vi "Calculate_Desired_Flowrates.vi"(8 "Strength (% by volume)":dbl=3.0 format="%.2f", 9 "Carrier_2 Q (l/min)":dbl=20.0 format="%.2f", 10 "Carrier_1 Q (l/min)":dbl=20.0 format="%.2f") -> (0 "Error Message":string, 1 "Trace Q l/min":dbl format="%.2f", 2 "Carrier 2 l/min":dbl format="%.2f", 3 "Carrier 1 l/min":dbl format="%.2f", 4 "Carrier Info":string)   [LabVIEW 2014]
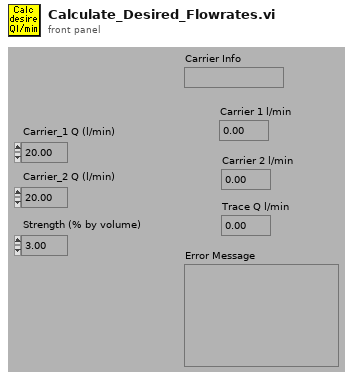
[diagram p1: front panel]
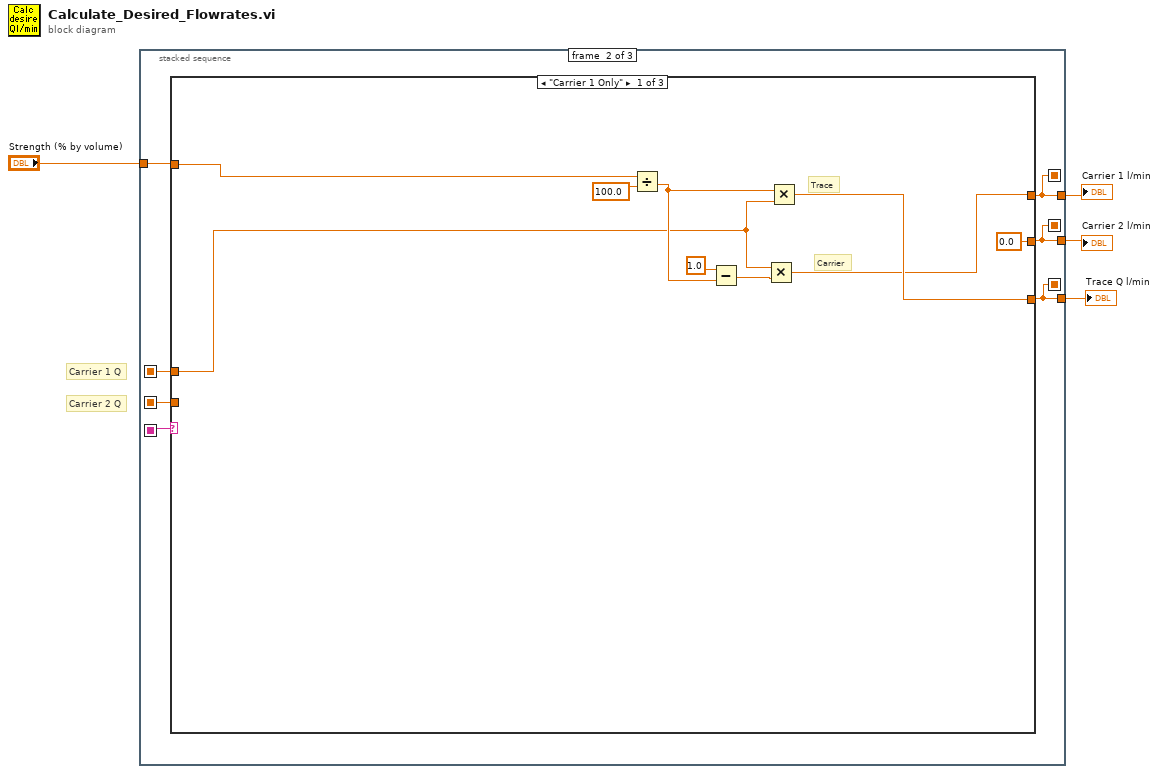
[diagram p0: block diagram]
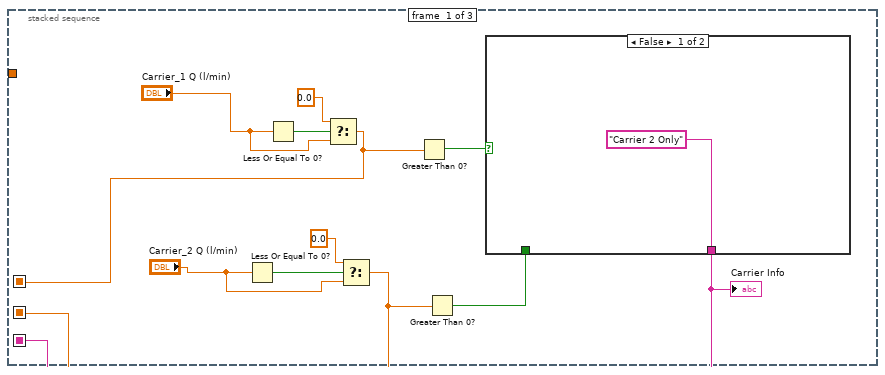
[diagram p2: hidden frame]
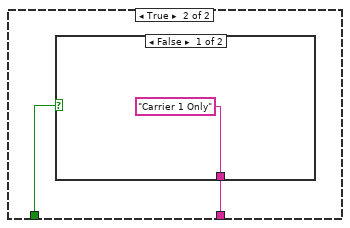
[diagram p3: hidden frame]
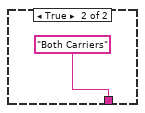
[diagram p4: hidden frame]
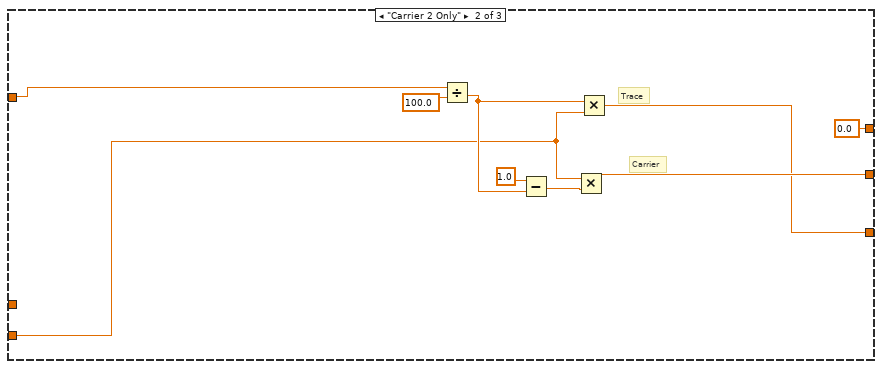
[diagram p5: hidden frame]
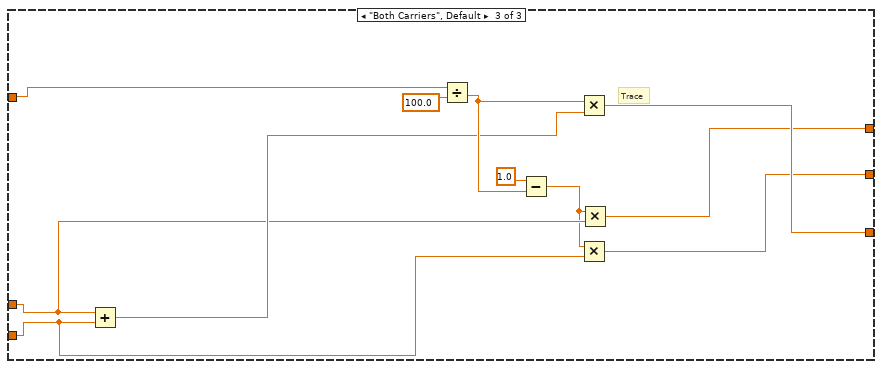
[diagram p6: hidden frame]
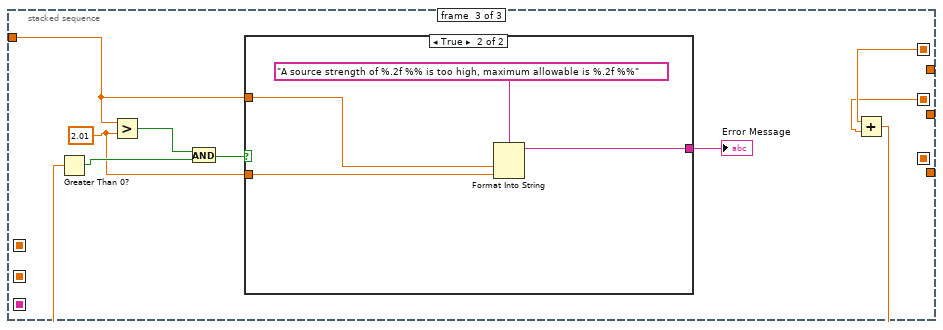
[diagram p7: hidden frame]
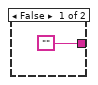
[diagram p8: hidden frame]
diagram:
  # "Carrier 2 Q"
  # "Carrier 1 Q"
  n1 = stacked-sequence {
    seq-local: [_ w24 _] -> [_ _ w60]
    seq-local: [_ w25 _] -> [_ _ w59]
    seq-local: [_ w26 _] -> [_ _ _]
    seq-local: [w9 _ _] -> [_ w22 _]
    seq-local: [w8 _ _] -> [_ w21 _]
    seq-local: [w5 _ _] -> [_ w23 _]
    tunnel: "Strength (% by volume)" -> [_ w27 w61]
    tunnel: [_ w26 _] -> w3
    tunnel: [_ w24 _] -> w2
    tunnel: [_ w25 _] -> w1
    frame #0 {
      n2 = Less Or Equal To 0?(x="Carrier_2 Q (l/min)") -> (x <= 0?=w11:bool)
      n3 = Less Or Equal To 0?(x="Carrier_1 Q (l/min)") -> (x <= 0?=w15:bool)
      n4 = Select(t=0.0, s=w15, f="Carrier_1 Q (l/min)") -> (s? t:f=w9:dbl)
      n5 = Select(t=0.0, s=w11, f="Carrier_2 Q (l/min)") -> (s? t:f=w8:dbl)
      n6 = Greater Than 0?(x=w9) -> (x > 0?=w7:bool)
      n7 = Greater Than 0?(x=w8) -> (x > 0?=w6:bool)
      n8 = case shown="False" w7 {
        tunnel: w6 -> [_ w18]
        tunnel: ["Carrier 2 Only" w17] -> w5
        frame False {
        }
        frame True {
          n9 = case shown="False" w18 {
            tunnel: ["Carrier 1 Only" "Both Carriers"] -> w17
            frame False {
            }
            frame True {
            }
          }
        }
      }
      "Carrier Info" <- w5
    }
    frame #1 {
      n10 = case shown="\"Carrier 1 Only\"" w23 {
        tunnel: w27 -> [w33 w41 w53]
        tunnel: [0.0 ("Qc2") w40 w46] -> w25
        tunnel: [w31 w39 w52] -> w26
        tunnel: [w30 0.0 ("Qc1") w47] -> w24
        tunnel: w22 -> [w28 _ w50]
        tunnel: w21 -> [_ w37 w48]
        frame "Carrier 1 Only" {
          # "Carrier"
          # "Trace"
          n11 = Divide(x=w33, y=100.0) -> (x/y=w32:dbl)
          n12 = Subtract(x=1.0, y=w32) -> (x-y=w36:dbl)
          n13 = Multiply(x=w28, y=w36) -> (x*y=w30:dbl)
          n14 = Multiply(x=w32, y=w28) -> (x*y=w31:dbl)
        }
        frame "Carrier 2 Only" {
          # "Carrier"
          # "Trace"
          n15 = Divide(x=w41, y=100.0) -> (x/y=w42:dbl)
          n16 = Subtract(x=1.0, y=w42) -> (x-y=w45:dbl)
          n17 = Multiply(x=w37, y=w45) -> (x*y=w40:dbl)
          n18 = Multiply(x=w42, y=w37) -> (x*y=w39:dbl)
        }
        frame "Both Carriers", Default {
          # "Trace"
          n19 = Add(x=w50, y=w48) -> (x+y=w51:dbl)
          n20 = Divide(x=w53, y=100.0) -> (x/y=w54:dbl)
          n21 = Subtract(x=1.0, y=w54) -> (x-y=w49:dbl)
          n22 = Multiply(x=w54, y=w51) -> (x*y=w52:dbl)
          n23 = Multiply(x=w49, y=w48) -> (x*y=w46:dbl)
          n24 = Multiply(x=w49, y=w50) -> (x*y=w47:dbl)
        }
      }
    }
    frame #2 {
      w62 = 2.01 ("y")
      n25 = Greater?(x=w61, y=w62) -> (0:w65:bool)
      n26 = Add(x=w60, y=w59) -> (x+y=w58:dbl)
      n27 = Greater Than 0?(x=w58) -> (x > 0?=w64:bool)
      n28 = And(x=w65, y=w64) -> (x .and. y?=w63:bool)
      n29 = case shown="True" w63 {
        tunnel: w61 -> [_ w70]
        tunnel: w62 -> [_ w68]
        tunnel: ["" w67] -> w57
        frame False {
        }
        frame True {
          n30 = Format Into String(format string="A source strength of %.2f %% is too high, maximum allowable is %.2f %%" ("Format String"), w70, w68) -> (resulting string=w67:string)  [unwired: 2 in, 1 out]
        }
      }
      "Error Message" <- w57
    }
  }
  "Carrier 1 l/min" <- w2
  "Carrier 2 l/min" <- w1
  "Trace Q l/min" <- w3
